vi "Write left SR.vi"(5 "left SR":refnum<class "LeftShiftRegister.lvclass">[](array[class]), 9 "ShiftRegister in":refnum<class "ShiftRegister.lvclass">) -> (3 "ShiftRegister out":refnum<class "ShiftRegister.lvclass">)   [LabVIEW 2014, in "Raspberry Pi Compatible Compiler for LabVIEW.lvlib" / "ShiftRegister.lvclass"]
uses:
  ShiftRegister.lvclass
  LeftShiftRegister/LeftShiftRegister.lvclass
  ShiftRegister.lvclass/ShiftRegister.ctl
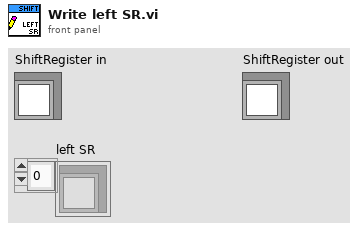
[diagram p1: front panel]
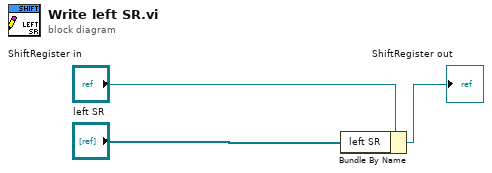
[diagram p0: block diagram]
diagram:
  n1 = Bundle By Name(cluster="ShiftRegister in", "left SR"="left SR") -> (→"ShiftRegister out":refnum<class "ShiftRegister.lvclass">)
